vi "Write Update Fan Status Message.vi"(10 "更新消息":refnum<class "Update Fan Status Msg.lvclass">, 11 "双风扇输入":refnum<class "Dual Fan.lvclass">) -> (3 "双风扇输出":refnum<class "Dual Fan.lvclass">)   [LabVIEW 2015, in "Dual Fan.lvlib" / "Dual Fan.lvclass"]
doc: "写入向调用方发送风扇状态更新的消息对象。调用方应在调用Launch Actor.vi之前设置该值。"
uses:
  Dual Fan.lvclass
  Update Fan Status Msg/Update Fan Status Msg.lvclass
  Dual Fan.lvclass/Dual Fan.ctl
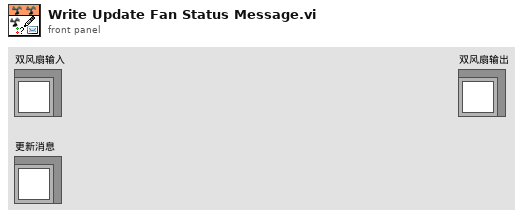
[diagram p1: front panel]
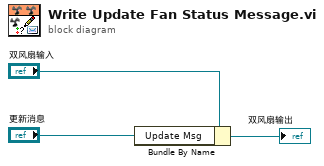
[diagram p0: block diagram]
diagram:
  n1 = Bundle By Name(cluster="双风扇输入", "Update Msg"="更新消息") -> (→"双风扇输出":refnum<class "Dual Fan.lvclass">)
